vi "Send Message.vi"(8 "error in (no error)":errorcluster, 9 "Data In":variant, 10 "Message String":string, 11 "Send to MsgQ":T1) -> (0 "error out":errorcluster)   [LabVIEW 2012]
uses:
  MsgQ Loops enum.ctl
  Common/Interloop MessageQ/Message que instance modes enum.ctl
  Main MsgQ.lvlib
  Common/Interloop MessageQ/Interloop MessageQ.lvlib
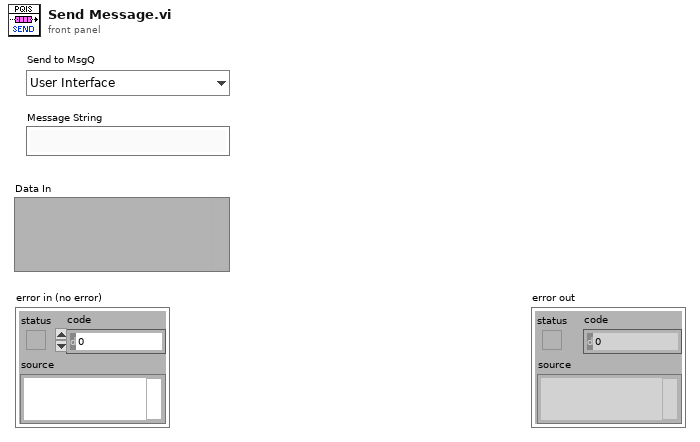
[diagram p1: front panel]
types:
  T1 = typedef "Main MsgQ.lvlib/MsgQ Loops enum.ctl" = enum16{"User Interface", "File IO", "DIO", "Camera 1", "Camera 2", "Camera 3", "Camera 4", "Analysis", "Keyboard"}
  T2 = typedef "Interloop MessageQ.lvlib/Message que instance modes enum.ctl" = enum16{"Initialize", "Broadcast Message", "Send Message", "Read Message", "Kill"}
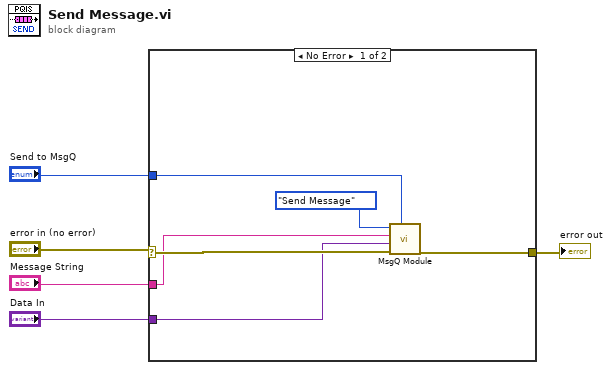
[diagram p0: block diagram]
diagram:
  n1 = case shown="No Error" "error in (no error)" {
    selector: "error in (no error)" -> [w10 w12]
    tunnel: [w11 w12] -> w4
    tunnel: "Send to MsgQ" -> [w9 _]
    tunnel: "Message String" -> [w8 _]
    tunnel: "Data In" -> [w6 _]
    frame No Error {
      n2 = call "MsgQ Module.vi"("MsgQ enum"=w9, "error in (no error)"=w10, "Message Send Parameters"=w6, "Message Send String"=w8, "Mode"=Message_que_instance_modes_enum."Send Message") -> ("error out"=w11:errorcluster)  [unwired: 6 out]
    }
    frame Error {
    }
  }
  "error out" <- w4
